vi "SGL-to-I16.vi"(11 "Range":sgl(slide) scale=-180.0..180.0) -> (1 "lo(x)":u8, 2 "hi(x)":u8, 3 "16bit integer":i16)   [LabVIEW 2017]
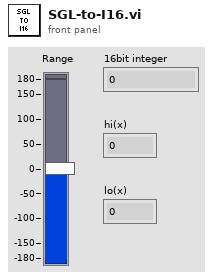
[diagram p1: front panel]
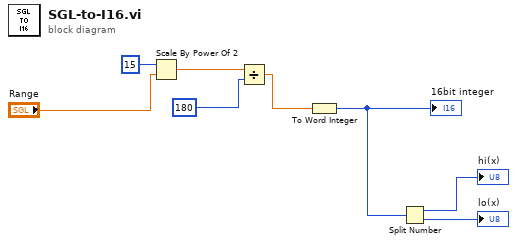
[diagram p0: block diagram]
diagram:
  n1 = Scale By Power Of 2(n=i16 15, x="Range") -> (x*2^n=w8:sgl)
  n2 = Divide(x=w8, y=u8 180) -> (x/y=w6:sgl)
  n3 = To Word Integer(number=w6) -> (16bit integer=w1:i16)
  "16bit integer" <- w1
  n4 = Split Number(x=w1) -> (hi(x)=→"hi(x)":u8, lo(x)=→"lo(x)":u8)
